vi "CMDCore.vi"(8 "error in (no error)":errorcluster caption="错误输入（无错误）", 11 "MainPage 输入":refnum<class "MainPage.lvclass">) -> (0 "error out":errorcluster caption="错误输出", 3 "MainPage 输出":refnum<class "MainPage.lvclass">)   [LabVIEW 2019, in "MainPage.lvlib" / "MainPage.lvclass"]
uses:
  MainPage.lvclass
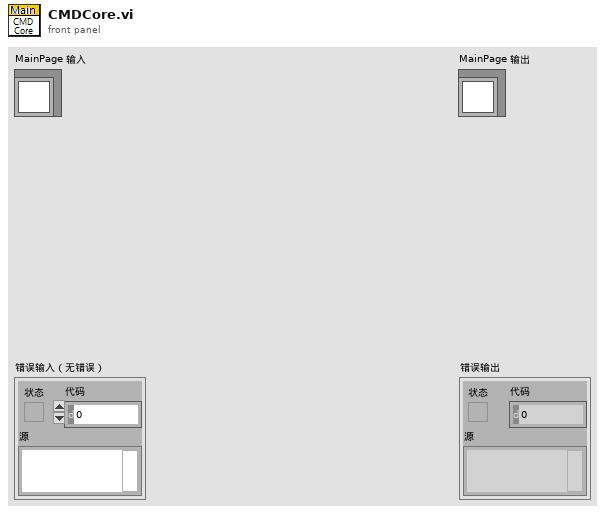
[diagram p1: front panel]
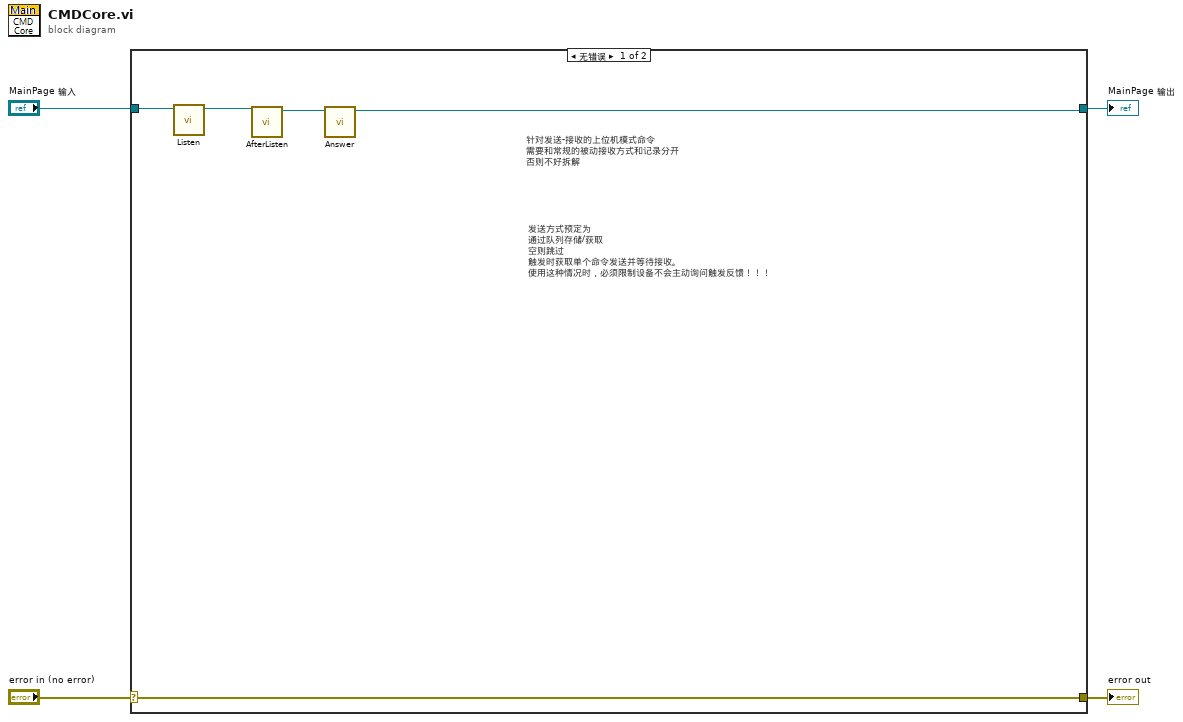
[diagram p0: block diagram]
diagram:
  n1 = case shown="无错误" "error in (no error)" {
    selector: "error in (no error)" -> [w9 w11]
    tunnel: [w9 w11] -> w3
    tunnel: [w5 w10] -> w1
    tunnel: "MainPage 输入" -> [w8 w10]
    frame No Error {
      # "发送方式预定为\n通过队列存储/获取\n空则跳过\n触发时获取单个命令发送并等待接收。\n使用这种情况时，必须限制设备不会主动询问触发反馈！！！"
      # "针对发送-接收的上位机模式命令\n需要和常规的被动接收方式和记录分开\n否则不好拆解"
      n2 = call-dynamic "Listen.vi"("MainPage 输入"=w8) -> ("MainPage 输出"=w7:refnum<class "MainPage.lvclass">)  [unwired: 9 in, 1 out]
      n3 = call-dynamic "AfterListen.vi"("MainPage 输入"=w7) -> ("MainPage 输出"=w6:refnum<class "MainPage.lvclass">)  [unwired: 9 in, 1 out]
      n4 = call-dynamic "Answer.vi"("MainPage 输入"=w6) -> ("MainPage 输出"=w5:refnum<class "MainPage.lvclass">)  [unwired: 9 in, 1 out]
    }
    frame Error {
    }
  }
  "error out" <- w3
  "MainPage 输出" <- w1
